vi "Prober_InitObject.vi"(8 "error in (no error)":errorcluster, 10 "Prober Configuration":variant, 11 "TeslaVeloxProbeStation in":refnum<class "TeslaVeloxProbeStation.lvclass">) -> (0 "error out":errorcluster, 3 "TeslaVeloxProbeStation out":refnum<class "TeslaVeloxProbeStation.lvclass">)   [LabVIEW 2018, in "TeslaVeloxProbeStation.lvclass"]
uses:
  TeslaVeloxProbeStation.lvclass
  TeslaVeloxProbeStation.lvclass/TeslaVeloxProbeStation.ctl
  TeslaVelox_GlobalConfig.vi
  Desktop/Kvasnicka/test_labview_library/Integration_toolkit_library/CascadeProbestation.lvlib
panel:
  out "ResourceName":string
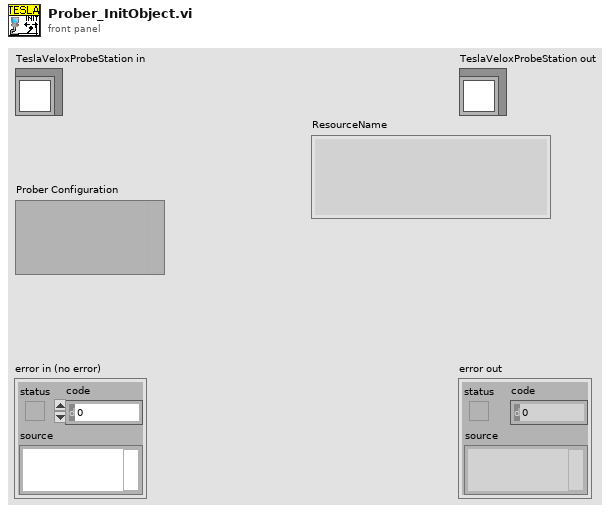
[diagram p1: front panel]
types:
  T1 = cluster{"IP address":string, "Separation gap[um]":dbl, "Port Number":i32, "Use Overdrive?":bool, "Touchdown method":enum16{"no feedback"}, "Coordinate system":enum16{"Cartesian", "X as index"}}
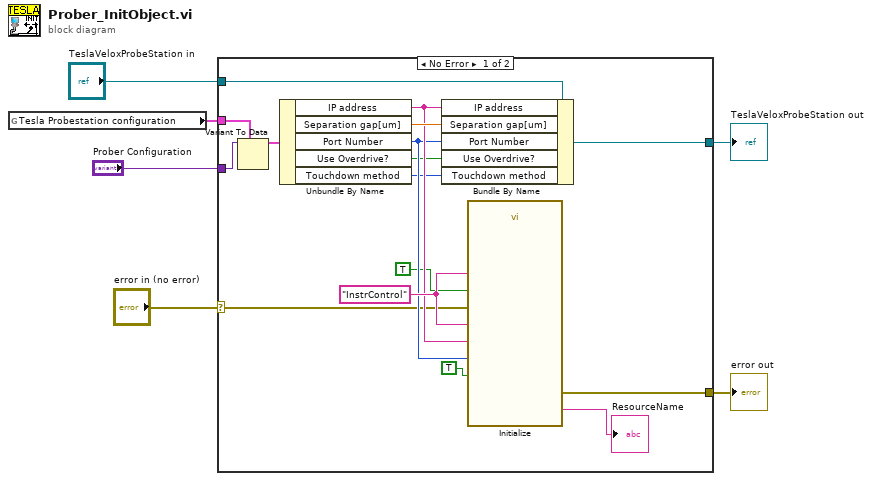
[diagram p0: block diagram]
diagram:
  n1 = global read "TeslaVelox_GlobalConfig.vi" "Tesla Probestation configuration"() -> (w1:T1)
  n2 = case shown="No Error" "error in (no error)" {
    selector: "error in (no error)" -> [w12 w24]
    tunnel: "Prober Configuration" -> [w22 _]
    tunnel: "TeslaVeloxProbeStation in" -> [w18 w23]
    tunnel: [w19 w23] -> w4
    tunnel: [w11 w24] -> w2
    tunnel: w1 -> [w7 _]
    frame No Error {
      w17 = "InstrControl" ("AppName")
      n3 = Variant To Data(type=w7, Variant=w22) -> (data=w21:T1)  [unwired: 1 in, 1 out]
      n4 = Unbundle By Name(w21) -> ("IP address"=w16:string, "Separation gap[um]"=w20:dbl, "Port Number"=w15:i32, "Use Overdrive?"=w9:bool, "Touchdown method"=w8:enum16{"no feedback"})
      n5 = Bundle By Name(cluster=w18, "IP address"=w16, "Separation gap[um]"=w20, "Port Number"=w15, "Use Overdrive?"=w9, "Touchdown method"=w8) -> (w19:refnum<class "TeslaVeloxProbeStation.lvclass">)
      n6 = call "Initialize.vi"("AppName"=w17, "IP Adress"=w16, "Port Number"=w15, "GroupName"=w17, "EnableNotification"=TRUE, "Use Socket Connection"=TRUE, "Error In (no error)"=w12) -> ("ResourceName"=→"ResourceName":string, "Error Out"=w11:errorcluster)  [unwired: 7 in]
    }
    frame Error {
    }
  }
  "error out" <- w2
  "TeslaVeloxProbeStation out" <- w4
